vi "change_old_color.vi"(7 "Parâmetros":T2={"Gyro Port"=0, "Sensor - Left"=3, "Sensor - Right"=3, "     Color \nSensor Port"=2, "Kp"=1, "Motor speed"=34, "Distance to street"=0.0, "Motor speed turns"=34} {"Color \nSensor Port" items=["Port 1", "Port 2", "Port 3", "Port 4"]; "Sensor - Right" items=["Port 1", "Port 2", "Port 3", "Port 4"]; "Sensor - Left" items=["Port 1", "Port 2", "Port 3", "Port 4"]; "Gyro Port" items=["Port 1", "Port 2", "Port 3", "Port 4"]}, 10 "NXT/EV3":T4) -> (2 "Detected Color":T3)   [LabVIEW 2016]
uses:
  <vilib>/NXT/Subs/LVHSConnector.ctl
  <vilib>/NXT/LegoClasses/BrickReference/BrickReference.lvclass
  <vilib>/NXT/Subs/ColorSensorColors.ctl
  <vilib>/NXT/Block Support/NXT_InputPort.ctl
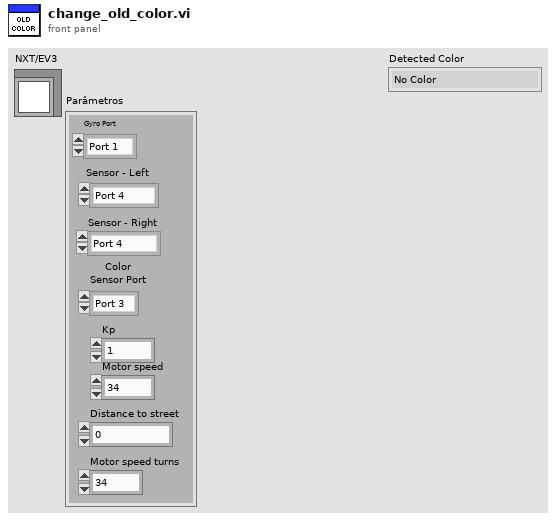
[diagram p1: front panel]
types:
  T1 = typedef "NXT_InputPort.ctl" = u32
  T2 = cluster{"Gyro Port":T1, "Sensor - Left":T1, "Sensor - Right":T1, "     Color \nSensor Port":T1, "Kp":i32, "Motor speed":i32, "Distance to street":dbl, "Motor speed turns":i32}
  T3 = typedef "ColorSensorColors.ctl" = enum16{"No Color", "Black", "Blue", "Green", "Yellow", "Red", "White", "Brown"}
  T4 = typedef "LVHSConnector.ctl" = refnum<class "BrickReference.lvclass">
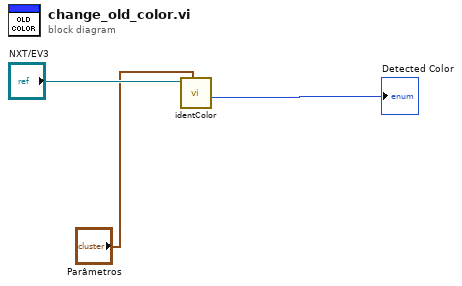
[diagram p0: block diagram]
diagram:
  n1 = call "identColor.vi"("Parâmetros"="Parâmetros", "NXT/EV3"="NXT/EV3") -> ("Collor"=→"Detected Color":T3)  [unwired: 9 in]
